vi "Initialize.vi"(8 "error in (no error)":errorcluster, 11 "S4ACS_GUI in":refnum<class "S4GUI.lvclass">) -> (0 "error out":errorcluster, 3 "S4ACS_GUI out":refnum<class "S4GUI.lvclass">)   [LabVIEW 2018, in "S4GUI.lvclass"]
uses:
  S4GUI.lvclass
  S4GUI.lvclass/S4GUI.ctl
  TCS/TCS.lvclass
  Instrument/Instrument.lvclass
  Acquisition/Acquisition.lvclass
  SyncBox/Sync Box.lvclass
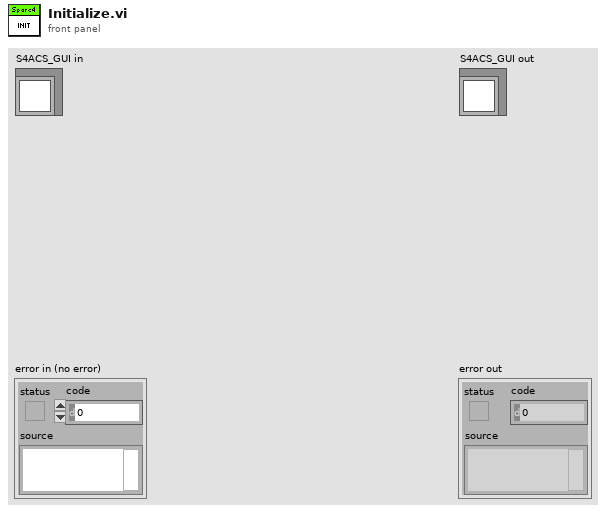
[diagram p1: front panel]
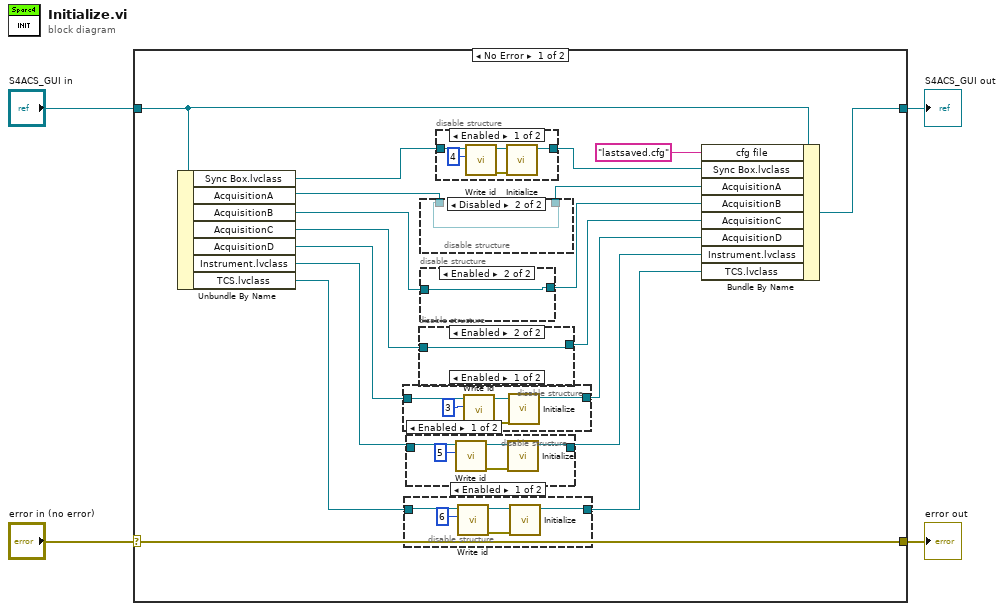
[diagram p0: block diagram]
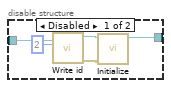
[diagram p3: hidden frame]
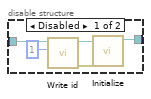
[diagram p6: hidden frame]
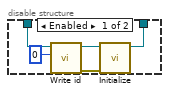
[diagram p7: hidden frame]
diagram:
  n1 = case shown="No Error" "error in (no error)" {
    selector: "error in (no error)" -> [w18 w66]
    tunnel: [w18 w66] -> w3
    tunnel: [w8 w65] -> w1
    tunnel: "S4ACS_GUI in" -> [w9 w65]
    frame No Error {
      n2 = Unbundle By Name(w9) -> ("Sync Box.lvclass"=w12:refnum<class "Sync Box.lvclass">, "AcquisitionA"=w20:refnum<class "Acquisition.lvclass">, "AcquisitionB"=w19:refnum<class "Acquisition.lvclass">, "AcquisitionC"=w17:refnum<class "Acquisition.lvclass">, "AcquisitionD"=w16:refnum<class "Acquisition.lvclass">, "Instrument.lvclass"=w11:refnum<class "Instrument.lvclass">, "TCS.lvclass"=w6:refnum<class "TCS.lvclass">)
      n3 = disable-structure shown="Enabled" {
        disable-tunnel: w16 -> [w27 w28]
        disable-tunnel: [w26 w28] -> w14
        frame Enabled {
          n4 = call-dynamic "Write id.vi"("id"=u32 3, "Server in"=w27) -> ("error out"=w23:errorcluster, "Server out"=w24:refnum<class "Acquisition.lvclass">)  [unwired: 8 in]
          n5 = call-dynamic "Initialize.vi"("error in (no error)"=w23, "Acquisition in"=w24) -> ("Acquisition out"=w26:refnum<class "Acquisition.lvclass">)  [unwired: 8 in, 1 out]
        }
        frame Disabled {
        }
      }
      n6 = disable-structure shown="Enabled" {
        disable-tunnel: w6 -> [w43 w46]
        disable-tunnel: [w42 w46] -> w5
        frame Enabled {
          n7 = call-dynamic "Write id.vi"("id"=u32 6, "Server in"=w43) -> ("error out"=w45:errorcluster, "Server out"=w44:refnum<class "TCS.lvclass">)  [unwired: 8 in]
          n8 = call-dynamic "Initialize.vi"("error in (no error)"=w45, "TCS in"=w44) -> ("TCS out"=w42:refnum<class "TCS.lvclass">)  [unwired: 8 in, 1 out]
        }
        frame Disabled {
        }
      }
      n9 = disable-structure shown="Enabled" {
        disable-tunnel: w11 -> [w36 w40]
        disable-tunnel: [w35 w40] -> w10
        frame Enabled {
          n10 = call-dynamic "Write id.vi"("id"=u32 5, "Server in"=w36) -> ("error out"=w37:errorcluster, "Server out"=w38:refnum<class "Instrument.lvclass">)  [unwired: 8 in]
          n11 = call-dynamic "Initialize.vi"("error in (no error)"=w37, "Instrument in"=w38) -> ("Instrument out"=w35:refnum<class "Instrument.lvclass">)  [unwired: 8 in, 1 out]
        }
        frame Disabled {
        }
      }
      n12 = disable-structure shown="Enabled" {
        disable-tunnel: w17 -> [w33 w34]
        disable-tunnel: [w32 w34] -> w15
        frame Disabled {
          n13 = call-dynamic "Write id.vi"("id"=u32 2, "Server in"=w33) -> ("error out"=w31:errorcluster, "Server out"=w30:refnum<class "Acquisition.lvclass">)  [unwired: 8 in]
          n14 = call-dynamic "Initialize.vi"("error in (no error)"=w31, "Acquisition in"=w30) -> ("Acquisition out"=w32:refnum<class "Acquisition.lvclass">)  [unwired: 8 in, 1 out]
        }
        frame Enabled {
        }
      }
      n15 = disable-structure shown="Disabled" {
        disable-tunnel: [w57 w58] -> w22
        disable-tunnel: w20 -> [w56 w58]
        frame Enabled {
          n16 = call-dynamic "Write id.vi"("id"=u32 0, "Server in"=w56) -> ("error out"=w53:errorcluster, "Server out"=w54:refnum<class "Acquisition.lvclass">)  [unwired: 8 in]
          n17 = call-dynamic "Initialize.vi"("error in (no error)"=w53, "Acquisition in"=w54) -> ("Acquisition out"=w57:refnum<class "Acquisition.lvclass">)  [unwired: 8 in, 1 out]
        }
        frame Disabled {
        }
      }
      n18 = disable-structure shown="Enabled" {
        disable-tunnel: [w51 w52] -> w21
        disable-tunnel: w19 -> [w50 w52]
        frame Disabled {
          n19 = call-dynamic "Write id.vi"("id"=u32 1, "Server in"=w50) -> ("error out"=w47:errorcluster, "Server out"=w49:refnum<class "Acquisition.lvclass">)  [unwired: 8 in]
          n20 = call-dynamic "Initialize.vi"("error in (no error)"=w47, "Acquisition in"=w49) -> ("Acquisition out"=w51:refnum<class "Acquisition.lvclass">)  [unwired: 8 in, 1 out]
        }
        frame Enabled {
        }
      }
      n21 = disable-structure shown="Enabled" {
        disable-tunnel: [w63 w64] -> w13
        disable-tunnel: w12 -> [w62 w64]
        frame Enabled {
          n22 = call-dynamic "Write id.vi"("id"=u32 4, "Server in"=w62) -> ("error out"=w59:errorcluster, "Server out"=w60:refnum<class "Sync Box.lvclass">)  [unwired: 8 in]
          n23 = call-dynamic "Initialize.vi"("error in (no error)"=w59, "Sync Box in"=w60) -> ("Sync Box out"=w63:refnum<class "Sync Box.lvclass">)  [unwired: 8 in, 1 out]
        }
        frame Disabled {
        }
      }
      n24 = Bundle By Name(cluster=w9, "cfg file"="lastsaved.cfg", "Sync Box.lvclass"=w13, "AcquisitionA"=w22, "AcquisitionB"=w21, "AcquisitionC"=w15, "AcquisitionD"=w14, "Instrument.lvclass"=w10, "TCS.lvclass"=w5) -> (w8:refnum<class "S4GUI.lvclass">)
    }
    frame Error {
    }
  }
  "error out" <- w3
  "S4ACS_GUI out" <- w1
